vi "FloatingPointComma.vi"(10 "Comma?":bool, 11 "String In":string) -> (1 "fixed":string, 3 "Numeric":dbl)   [LabVIEW 2022 SP3]
panel:
  out "number of replacements":i32
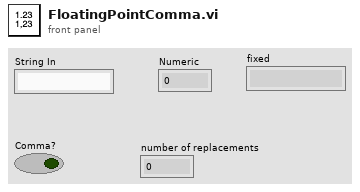
[diagram p1: front panel]
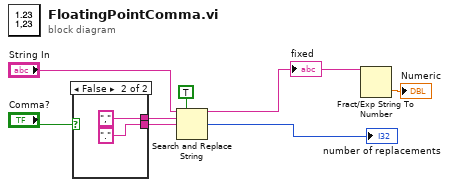
[diagram p0: block diagram]
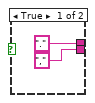
[diagram p2: hidden frame]
diagram:
  n1 = case shown="False" "Comma?" {
    tunnel: ["." ("search string") "," ("search string")] -> w7
    tunnel: ["," ("replace string (\"\")") "." ("replace string (\"\")")] -> w6
    frame True {
    }
    frame False {
    }
  }
  n2 = Search and Replace String(replace all?=TRUE ("replace all? (F)"), input string="String In", search string=w7, replace string=w6) -> (result string=w2:string, number of replacements=→"number of replacements":i32)  [unwired: 4 in, 2 out]
  "fixed" <- w2
  n3 = Fract/Exp String To Number(string=w2) -> (number=→"Numeric":dbl)  [unwired: 3 in, 1 out]
